vi "TDMS_Viewer.vi"() -> ()   [LabVIEW 2012]
panel:
  in  "TDMS file path":path
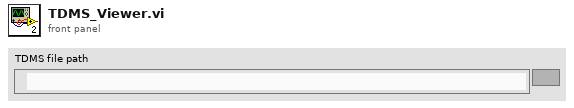
[diagram p1: front panel]
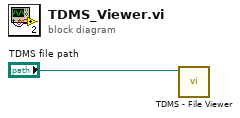
[diagram p0: block diagram]
diagram:
  n1 = call <vilib>:"TDMS - File Viewer.vi"("file path"="TDMS file path") -> ()  [unwired: 5 in, 2 out]
